vi "LoadControlPanel.vi"(8 "error in (no error)":errorcluster, 10 "Actor In":refnum<class "Actor.lvclass">, 11 "Camera_Prime95B in":refnum<class "Camera_Prime95B.lvclass">) -> (0 "error out":errorcluster, 3 "Camera_Prime95B out":refnum<class "Camera_Prime95B.lvclass">)   [LabVIEW 2020, in "Camera_Prime95B.lvlib" / "Camera_Prime95B.lvclass"]
uses:
  Camera_Prime95B.lvclass
  <vilib>/ActorFramework/Actor/Actor.lvclass
  ViewController/Prime95BCameraController/CameraController.lvclass
  C:/Program Files/National Instruments/LabVIEW 2020/vi.lib/ActorFramework/Actor/Actor.lvclass
  Hardware Abstraction Layer/Component/Device/Device/DataExchange.ctl
  Hardware Abstraction Layer/Component/Camera/Camera/Camera.lvclass
  Interface/DataListener/DataListener.lvclass
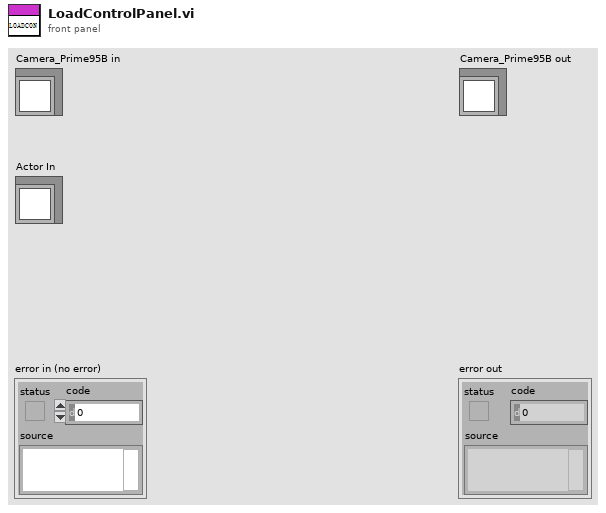
[diagram p1: front panel]
types:
  T1 = typedef "DataListener.lvclass/DataExchange.ctl" = cluster{"Source":string, "Destination":string, "Description":string, "value":variant}
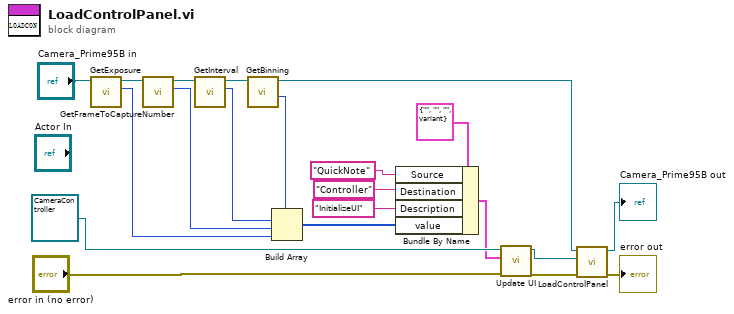
[diagram p0: block diagram]
diagram:
  n1 = call-dynamic "GetExposure.vi"("Camera in"="Camera_Prime95B in") -> ("Setting.Exposure"=w1:i32, "Camera out"=w16:refnum<class "Camera_Prime95B.lvclass">)  [unwired: 8 in, 1 out]
  n2 = call-dynamic "GetFrameToCaptureNumber.vi"("Camera in"=w16) -> ("Setting.FramesToCapture"=w2:i32, "Camera out"=w17:refnum<class "Camera_Prime95B.lvclass">)  [unwired: 8 in, 1 out]
  n3 = call-dynamic "GetInterval.vi"("Camera in"=w17) -> ("Setting.Interval"=w3:i32, "Camera out"=w14:refnum<class "Camera_Prime95B.lvclass">)  [unwired: 8 in, 1 out]
  n4 = call-dynamic "GetBinning.vi"("Camera in"=w14) -> ("Setting.Binning.BinY"=w5:i32, "Camera out"=w15:refnum<class "Camera_Prime95B.lvclass">)  [unwired: 7 in, 2 out]
  n5 = Build Array(w5, w3, w2, w1) -> (w4:i32[])
  n6 = Bundle By Name(cluster=T1 {"Source"="", "Destination"="", "Description"="", "value"=variant} ("DataExchange"), "Source"="QuickNote", "Destination"="Controller", "Description"="InitializeUI", "value"=w4) -> (w6:T1)
  n7 = call-dynamic "Update UI.vi"("error in (no error)"="error in (no error)", "DataExchange"=w6, "Camera Prime95B Controller in"=refnum<class "CameraController.lvclass"> refnum ("Prime95BCameraController.lvlib:Prime95BCameraController.lvclass")) -> ("error out"=w13:errorcluster, "Camera Prime95B Controller out"=w11:refnum<class "CameraController.lvclass">)  [unwired: 7 in]
  n8 = call-parent "LoadControlPanel.vi"("error in (no error)"=w13, "Actor In"=w11, "GRMActor in"=w15) -> ("error out"=→"error out":errorcluster, "GRMActor out"=→"Camera_Prime95B out":refnum<class "Camera_Prime95B.lvclass">)  [unwired: 7 in]
